vi "write front panel string control.vi"(0 "VI Ref":refnum<vi>, 5 "string":string, 7 "control label":string, 11 "error in":errorcluster) -> (4 "dup VI Ref":refnum<vi>, 15 "error out":errorcluster)   [LabVIEW 2020]
uses:
  <vilib>/Utility/traverseref.llb/TRef TravTarget.ctl
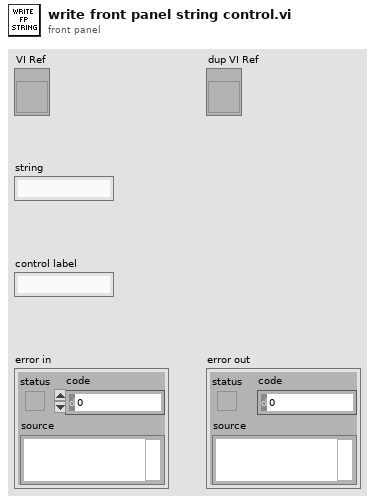
[diagram p1: front panel]
types:
  T1 = typedef "TRef TravTarget.ctl" = enum16{"FP", "BD", "Other"}
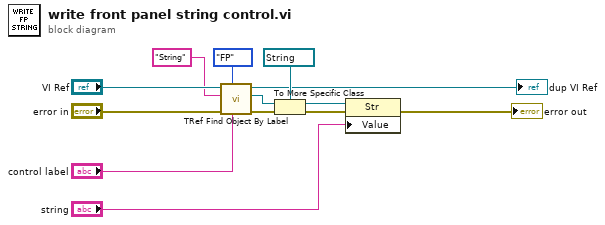
[diagram p0: block diagram]
diagram:
  n1 = call <vilib>:"TRef Find Object By Label.vi"("Label"="control label", "Traverse Target"=TRef_TravTarget."FP", "error in (no error)"="error in", "Class Name"="String", "VI Ref"="VI Ref") -> ("error out"=w10:errorcluster, "Found Obj Ref"=w7:refnum<vi>, "dup VI Ref"=→"dup VI Ref":refnum<vi>)  [unwired: 3 in, 1 out]
  n2 = To More Specific Class(target class=refnum<vi> refnum ("Other Refnum"), reference=w7, error in=w10) -> (specific class reference=w9:refnum<vi>, error out=w11:errorcluster)
  n3 = property class="Str"(reference=w9, error in=w11, "Value"="string") -> (error out=→"error out":errorcluster)  [unwired: 1 out]
